vi "Updater Convert TDMS Test Runs 4.3 to 5.0 PIM.vi"(7 "Source TDMS File In":refnum<k34>, 8 "error in (no error)":errorcluster, 10 "Group Name In":string, 11 "New TDMS File In":refnum<k34>) -> (0 "error out":errorcluster, 2 "Group Name Out":string, 3 "New TDMS File Out":refnum<k34>, 5 "Source TDMS File Out":refnum<k34>)   [LabVIEW 2011]
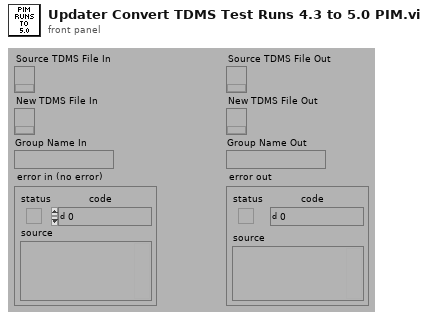
[diagram p1: front panel]
types:
  T1 = typedef "PIM Channel Type.ctl" = enum16{"Invalid", "Frequency", "Power", "CheckTx", "Unleveled", "Squelch", "Time", "Ref Limit", "IM Overload", "IM Power", "IM Frequency"}
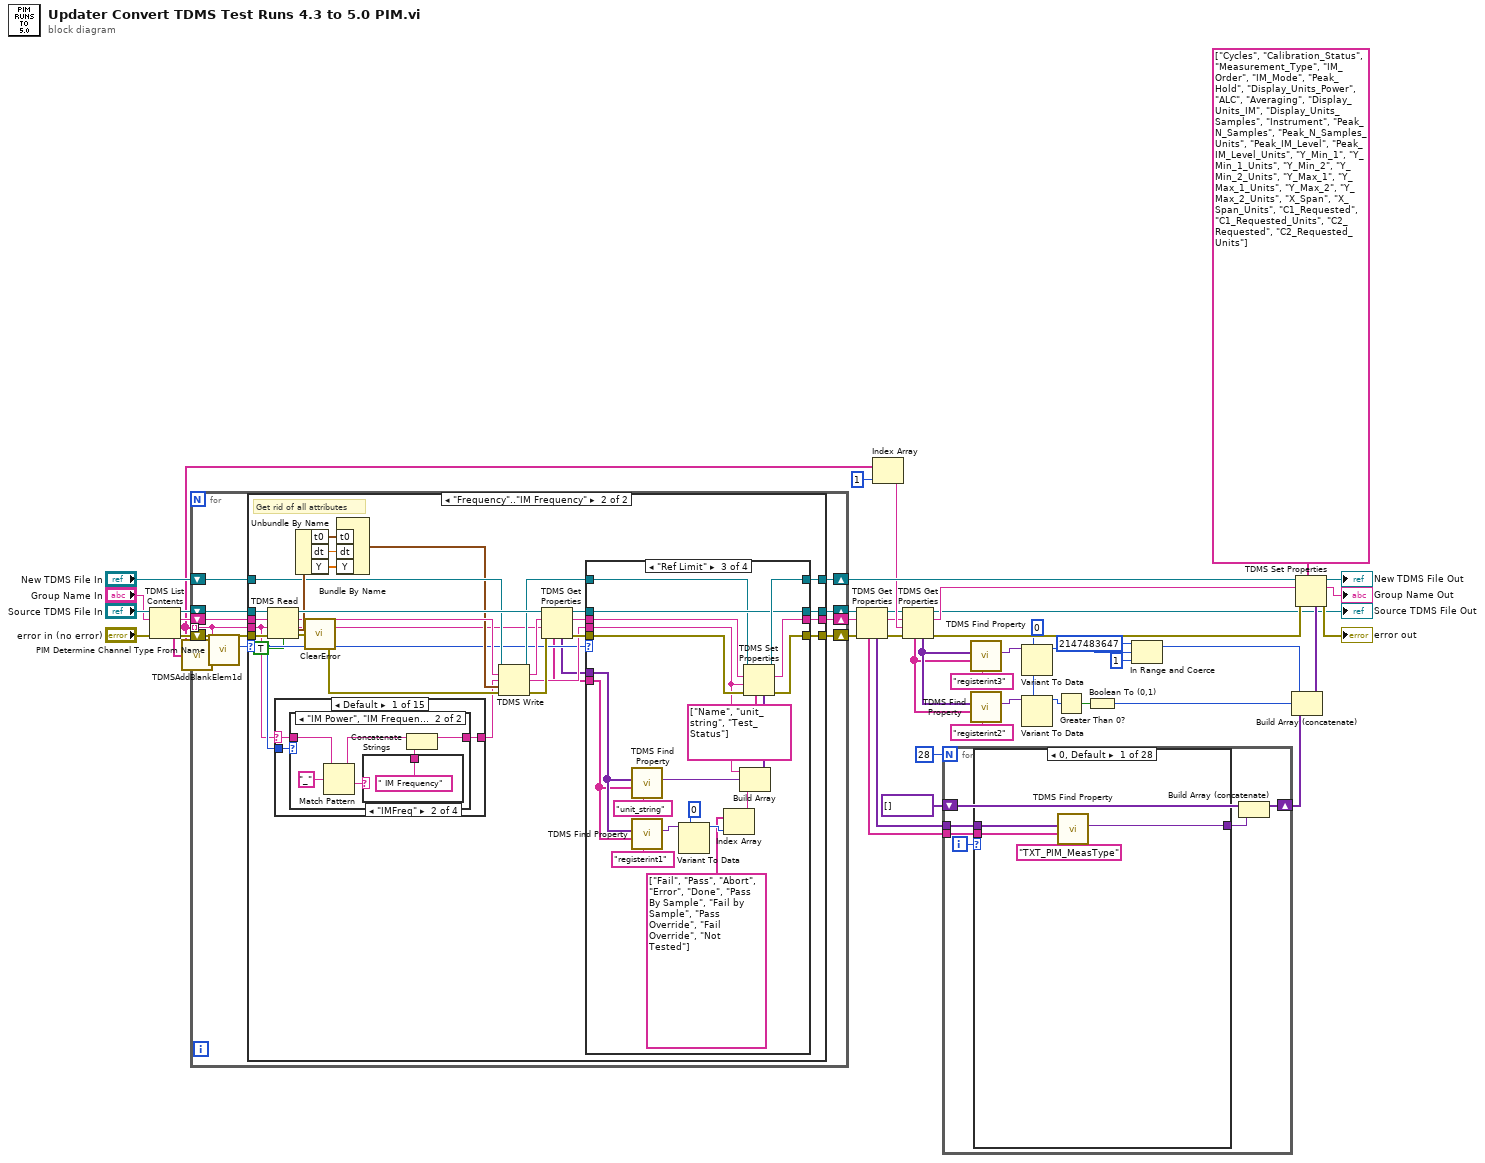
[diagram p0: block diagram]
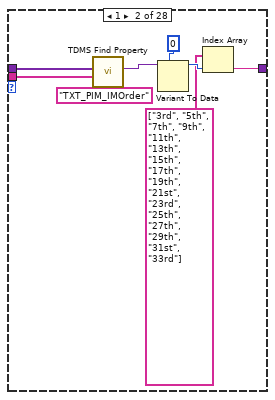
[diagram p2: hidden frame]
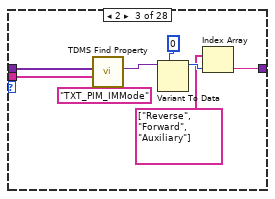
[diagram p3: hidden frame]
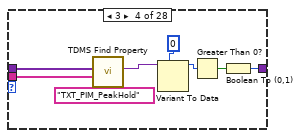
[diagram p4: hidden frame]
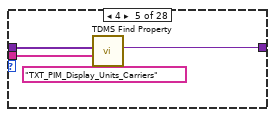
[diagram p5: hidden frame]
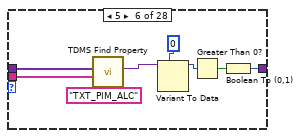
[diagram p6: hidden frame]
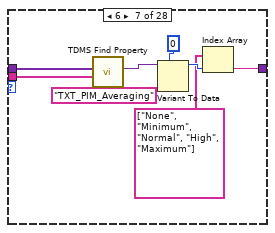
[diagram p7: hidden frame]
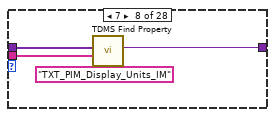
[diagram p8: hidden frame]
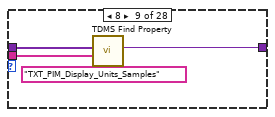
[diagram p9: hidden frame]
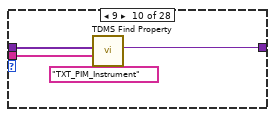
[diagram p10: hidden frame]
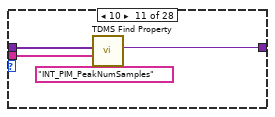
[diagram p11: hidden frame]
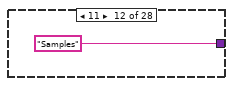
[diagram p12: hidden frame]
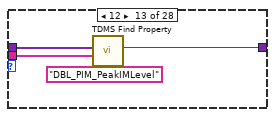
[diagram p13: hidden frame]
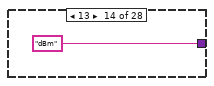
[diagram p14: hidden frame]
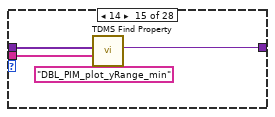
[diagram p15: hidden frame]
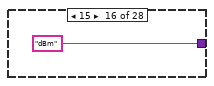
[diagram p16: hidden frame]
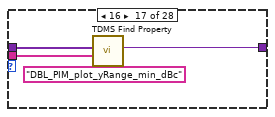
[diagram p17: hidden frame]
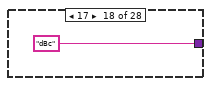
[diagram p18: hidden frame]
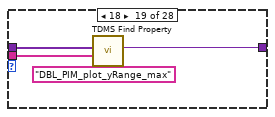
[diagram p19: hidden frame]
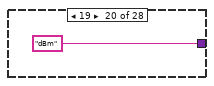
[diagram p20: hidden frame]
diagram:
  w18 = 0
  n1 = TDMS List Contents(4:"error in (no error)", 6:"Group Name In", 7:"Source TDMS File In") -> (0:w42:errorcluster, 1:w1:string[], 2:w40:string, 3:w41:refnum<k34>)
  n2 = call <vilib>:"TDMSAddBlankElem1d.vi"("input string array"=w1) -> ("output string array with blank element at the beginning"=w14:string[])
  n3 = for {
    shift-right: [w54] -> w11
    shift-left: w42 -> [w51]
    shift-right: [w55] -> w12
    shift-left: w41 -> [w50]
    tunnel: w14 -> [w48] mode=indexing
    shift-right: [w53] -> w10
    shift-left: w40 -> [w49]
    shift-right: [w52] -> w30
    shift-left: "New TDMS File In" -> [w47]
    n4 = call "PIM Determine Channel Type From Name.vi"("Channel Name"=w48) -> ("Channel Type"=w46:T1)  [unwired: 10 out]
    n5 = case shown="\"Frequency\"..\"IM Frequency\"" w46 {
      selector: w46 -> [_ w66]
      tunnel: [w59 w90] -> w55
      tunnel: [w56 w89] -> w54
      tunnel: [w58 w88] -> w53
      tunnel: [w57 w87] -> w52
      tunnel: w51 -> [w56 w83]
      tunnel: w50 -> [w59 w81]
      tunnel: w49 -> [w58 w80]
      tunnel: w48 -> [_ w65]
      tunnel: w47 -> [w57 w75]
      frame "Invalid" {
        # "Empty channel for Group level."
      }
      frame "Frequency".."IM Frequency" {
        # "Get rid of all attributes"
        n6 = TDMS Read(0:w81, 5:w80, 7:w65, 11:w83, 13:TRUE ("return channels in file order? (F)")) -> (4:w82:refnum<k34>, 6:w73:string, 8:w68:string, 10:w79:waveform(dbl), 15:w61:errorcluster)  [unwired: 3 in, 1 out]
        n7 = case shown="Default" w65 {
          selector: w65 -> [w92 _ _ _ _ _ _ _ _ _ _ _ _ _ _]
          tunnel: [w91 "Tx1 Frequency" "Tx1 Power" "Tx1 CheckTx" "Tx1 Unleveled" "Tx1 Squelch" "Tx2 Frequency" "Tx2 Power" "Tx2 CheckTx" "Tx2 Unleveled" "Tx2 Squelch" "Elapsed Time" "Ref Limit 1" "Ref Limit 2" "IM Overload"] -> w64
          tunnel: w66 -> [w93 _ _ _ _ _ _ _ _ _ _ _ _ _ _]
          frame Default {
            n8 = case shown="\"IM Power\", \"IM Frequency\"" w93 {
              tunnel: w92 -> [w94 w99]
              tunnel: [w94 w95] -> w91
              frame Default {
              }
              frame "IM Power", "IM Frequency" {
                n9 = Match Pattern(string=w99, regular expression="_") -> (before substring=w98:string, after substring=w97:string)  [unwired: 3 out]
                n10 = case shown="\"IMFreq\"" w97 {
                  tunnel: [_ " IM Frequency" " IM Power 1" " IM Power 2"] -> w96
                  frame Default {
                  }
                  frame "IMFreq" {
                  }
                  frame "IMPower" {
                  }
                  frame "IMPowerdBc" {
                  }
                }
                n11 = Concatenate Strings(w98, w96) -> (w95:string)
              }
            }
          }
          frame "Tx1Frequency" {
          }
          frame "Tx1Power" {
          }
          frame "Tx1CheckTx" {
          }
          frame "Tx1Unleveled" {
          }
          frame "Tx1Squelch" {
          }
          frame "Tx2Frequency" {
          }
          frame "Tx2Power" {
          }
          frame "Tx2CheckTx" {
          }
          frame "Tx2Unleveled" {
          }
          frame "Tx2Squelch" {
          }
          frame "elapsed_time" {
          }
          frame "RefLimit" {
          }
          frame "RefLimitdBc" {
          }
          frame "IMOverload" {
          }
        }
        n12 = Unbundle By Name(w79) -> ("t0"=w78:timestamp, "dt"=w77:dbl, "Y"=w76:dbl[])
        n13 = call <vilib>:"ClearError.vi"("error in (no error)"=w61) -> ("error out"=w74:errorcluster)
        n14 = Bundle By Name("t0"=w78, "dt"=w77, "Y"=w76) -> (w69:waveform(dbl))  [unwired: 1 out]
        n15 = TDMS Write(0:w75, 5:w73, 7:w64, 9:w69, 11:w74) -> (4:w70:refnum<k34>, 6:w72:string, 8:w67:string, 15:w71:errorcluster)  [unwired: 1 in]
        n16 = TDMS Get Properties(8:w71, 9:w68, 10:w72, 11:w82) -> (0:w86:errorcluster, 2:w85:string, 3:w84:refnum<k34>, 4:w63:variant[], 6:w62:string[])  [unwired: 3 out]
        n17 = case shown="\"Ref Limit\"" w66 {
          tunnel: w86 -> [w120 w124 w146 w158]
          tunnel: w85 -> [w119 w125 w147 w159]
          tunnel: w84 -> [w121 w130 w150 w161]
          tunnel: [w121 w130 w150 w161] -> w90
          tunnel: [w120 w133 w153 w162] -> w89
          tunnel: w67 -> [_ w122 w144 w157]
          tunnel: [w119 w134 w154 w163] -> w88
          tunnel: w70 -> [w118 w126 w148 w160]
          tunnel: [w118 w135 w155 w164] -> w87
          tunnel: w62 -> [_ w127 w141 _]
          tunnel: w63 -> [_ w128 w142 _]
          frame "Invalid" {
          }
          frame "Frequency", "Power", "Time", "IM Power", "IM Frequency" {
            n18 = call "TDMS Find Property.vi"("Property Name"="unit_string", "Property Names"=w127, "Property Values"=w128) -> ("Property Value"=w123:variant)  [unwired: 5 out]
            n19 = Build Array(w122, w123) -> (w131:variant[])
            n20 = TDMS Set Properties(5:w131, 7:string[] ["Name", "unit_string"], 8:w124, 9:w122, 10:w125, 11:w126) -> (0:w133:errorcluster, 2:w134:string, 3:w135:refnum<k34>)  [unwired: 1 out]
          }
          frame "Ref Limit" {
            n21 = call "TDMS Find Property.vi"("Property Name"="unit_string", "Property Names"=w141, "Property Values"=w142) -> ("Property Value"=w145:variant)  [unwired: 5 out]
            n22 = call "TDMS Find Property.vi"("Property Name"="registerint1", "Property Names"=w141, "Property Values"=w142) -> ("Property Value"=w137:variant)  [unwired: 5 out]
            n23 = Variant To Data(type=0, Variant=w137) -> (data=w140:i32)  [unwired: 1 in, 1 out]
            n24 = Index Array(array=string[] ["Fail", "Pass", "Abort", "Error", "Done", "Pass By Sample", "Fail by Sample", "Pass Override", "Fail Override", "Not Tested"], index=w140) -> (element=w136:string)
            n25 = Build Array(w144, w145, w136) -> (w151:variant[])
            n26 = TDMS Set Properties(5:w151, 7:string[] ["Name", "unit_string", "Test_Status"], 8:w146, 9:w144, 10:w147, 11:w148) -> (0:w153:errorcluster, 2:w154:string, 3:w155:refnum<k34>)  [unwired: 1 out]
          }
          frame "CheckTx".."Squelch", "IM Overload" {
            n27 = TDMS Set Properties(5:w157, 7:"Name", 8:w158, 9:w157, 10:w159, 11:w160) -> (0:w162:errorcluster, 2:w163:string, 3:w164:refnum<k34>)  [unwired: 1 out]
          }
        }
      }
    }
  }
  n28 = TDMS Get Properties(8:w11, 10:w10, 11:w12) -> (0:w8:errorcluster, 2:w7:string, 3:w9:refnum<k34>, 4:w4:variant[], 6:w3:string[])  [unwired: 1 in, 3 out]
  n29 = Index Array(array=w14, index=1) -> (element=w13:string)
  n30 = TDMS Get Properties(8:w8, 9:w13, 10:w7, 11:w9) -> (0:w39:errorcluster, 2:w36:string, 3:→"Source TDMS File Out":refnum<k34>, 4:w21:variant[], 6:w20:string[])  [unwired: 1 in, 2 out]
  n31 = for {
    N: 28 -> [_]
    shift-right: [w165] -> w2
    shift-left: variant[] [] ("appended array") -> [w166]
    tunnel: w4 -> [w169]
    tunnel: w3 -> [w168]
    i -> [w170]
    n32 = case shown="0, Default" w170 {
      tunnel: w169 -> [w173 w181 w189 w197 w201 w209 w217 w221 w225 w229 w233 _ w238 _ w243 _ w248 _ w253 _ w258 _ w263 _ w268 _ w273 _]
      tunnel: w168 -> [w172 w180 w188 w196 w200 w208 w216 w220 w224 w228 w232 _ w237 _ w242 _ w247 _ w252 _ w257 _ w262 _ w267 _ w272 _]
      tunnel: [w171 w175 w183 w192 w199 w204 w211 w219 w223 w227 w231 "Samples" w236 "dBm" w241 "dBm" w246 "dBc" w251 "dBm" w256 "dBc" w261 "MHz" w266 "dBm" w271 "dBm"] -> w167
      frame 0, Default {
        n33 = call "TDMS Find Property.vi"("Property Name"="TXT_PIM_MeasType", "Property Names"=w172, "Property Values"=w173) -> ("Property Value"=w171:variant)  [unwired: 5 out]
      }
      frame 1 {
        n34 = call "TDMS Find Property.vi"("Property Name"="TXT_PIM_IMOrder", "Property Names"=w180, "Property Values"=w181) -> ("Property Value"=w178:variant)  [unwired: 5 out]
        n35 = Variant To Data(type=0, Variant=w178) -> (data=w177:i32)  [unwired: 1 in, 1 out]
        n36 = Index Array(array=string[] ["3rd", "5th", "7th", "9th", "11th", "13th", "15th", "17th", "19th", "21st", "23rd", "25th", "27th", "29th", "31st", "33rd"], index=w177) -> (element=w175:string)
      }
      frame 2 {
        n37 = call "TDMS Find Property.vi"("Property Name"="TXT_PIM_IMMode", "Property Names"=w188, "Property Values"=w189) -> ("Property Value"=w186:variant)  [unwired: 5 out]
        n38 = Variant To Data(type=0, Variant=w186) -> (data=w185:i32)  [unwired: 1 in, 1 out]
        n39 = Index Array(array=string[] ["Reverse", "Forward", "Auxiliary"], index=w185) -> (element=w183:string)
      }
      frame 3 {
        n40 = call "TDMS Find Property.vi"("Property Name"="TXT_PIM_PeakHold", "Property Names"=w196, "Property Values"=w197) -> ("Property Value"=w194:variant)  [unwired: 5 out]
        n41 = Variant To Data(type=0, Variant=w194) -> (data=w191:i32)  [unwired: 1 in, 1 out]
        n42 = Greater Than 0?(x=w191) -> (x > 0?=w193:bool)
        n43 = Boolean To (0,1)(Boolean=w193) -> (0, 1=w192:i16)
      }
      frame 4 {
        n44 = call "TDMS Find Property.vi"("Property Name"="TXT_PIM_Display_Units_Carriers", "Property Names"=w200, "Property Values"=w201) -> ("Property Value"=w199:variant)  [unwired: 5 out]
      }
      frame 5 {
        n45 = call "TDMS Find Property.vi"("Property Name"="TXT_PIM_ALC", "Property Names"=w208, "Property Values"=w209) -> ("Property Value"=w206:variant)  [unwired: 5 out]
        n46 = Variant To Data(type=0, Variant=w206) -> (data=w203:i32)  [unwired: 1 in, 1 out]
        n47 = Greater Than 0?(x=w203) -> (x > 0?=w205:bool)
        n48 = Boolean To (0,1)(Boolean=w205) -> (0, 1=w204:i16)
      }
      frame 6 {
        n49 = call "TDMS Find Property.vi"("Property Name"="TXT_PIM_Averaging", "Property Names"=w216, "Property Values"=w217) -> ("Property Value"=w214:variant)  [unwired: 5 out]
        n50 = Variant To Data(type=0, Variant=w214) -> (data=w213:i32)  [unwired: 1 in, 1 out]
        n51 = Index Array(array=string[] ["None", "Minimum", "Normal", "High", "Maximum"], index=w213) -> (element=w211:string)
      }
      frame 7 {
        n52 = call "TDMS Find Property.vi"("Property Name"="TXT_PIM_Display_Units_IM", "Property Names"=w220, "Property Values"=w221) -> ("Property Value"=w219:variant)  [unwired: 5 out]
      }
      frame 8 {
        n53 = call "TDMS Find Property.vi"("Property Name"="TXT_PIM_Display_Units_Samples", "Property Names"=w224, "Property Values"=w225) -> ("Property Value"=w223:variant)  [unwired: 5 out]
      }
      frame 9 {
        n54 = call "TDMS Find Property.vi"("Property Name"="TXT_PIM_Instrument", "Property Names"=w228, "Property Values"=w229) -> ("Property Value"=w227:variant)  [unwired: 5 out]
      }
      frame 10 {
        n55 = call "TDMS Find Property.vi"("Property Name"="INT_PIM_PeakNumSamples", "Property Names"=w232, "Property Values"=w233) -> ("Property Value"=w231:variant)  [unwired: 5 out]
      }
      frame 11 {
      }
      frame 12 {
        n56 = call "TDMS Find Property.vi"("Property Name"="DBL_PIM_PeakIMLevel", "Property Names"=w237, "Property Values"=w238) -> ("Property Value"=w236:variant)  [unwired: 5 out]
      }
      frame 13 {
      }
      frame 14 {
        n57 = call "TDMS Find Property.vi"("Property Name"="DBL_PIM_plot_yRange_min", "Property Names"=w242, "Property Values"=w243) -> ("Property Value"=w241:variant)  [unwired: 5 out]
      }
      frame 15 {
      }
      frame 16 {
        n58 = call "TDMS Find Property.vi"("Property Name"="DBL_PIM_plot_yRange_min_dBc", "Property Names"=w247, "Property Values"=w248) -> ("Property Value"=w246:variant)  [unwired: 5 out]
      }
      frame 17 {
      }
      frame 18 {
        n59 = call "TDMS Find Property.vi"("Property Name"="DBL_PIM_plot_yRange_max", "Property Names"=w252, "Property Values"=w253) -> ("Property Value"=w251:variant)  [unwired: 5 out]
      }
      frame 19 {
      }
      frame 20 {
        n60 = call "TDMS Find Property.vi"("Property Name"="DBL_PIM_plot_yRange_max_dBc", "Property Names"=w257, "Property Values"=w258) -> ("Property Value"=w256:variant)  [unwired: 5 out]
      }
      frame 21 {
      }
      frame 22 {
        n61 = call "TDMS Find Property.vi"("Property Name"="DBL_PIM_plot_xRange_span", "Property Names"=w262, "Property Values"=w263) -> ("Property Value"=w261:variant)  [unwired: 5 out]
      }
      frame 23 {
      }
      frame 24 {
        n62 = call "TDMS Find Property.vi"("Property Name"="DBL_PIM_C1_Requested_dBm", "Property Names"=w267, "Property Values"=w268) -> ("Property Value"=w266:variant)  [unwired: 5 out]
      }
      frame 25 {
      }
      frame 26 {
        n63 = call "TDMS Find Property.vi"("Property Name"="DBL_PIM_C2_Requested_dBm", "Property Names"=w272, "Property Values"=w273) -> ("Property Value"=w271:variant)  [unwired: 5 out]
      }
      frame 27 {
      }
    }
    n64 = Build Array (concatenate)(w166, w167) -> (w165:variant[])
  }
  n65 = call "TDMS Find Property.vi"("Property Name"="registerint3", "Property Names"=w20, "Property Values"=w21) -> ("Property Value"=w28:variant)  [unwired: 5 out]
  n66 = call "TDMS Find Property.vi"("Property Name"="registerint2", "Property Names"=w20, "Property Values"=w21) -> ("Property Value"=w19:variant)  [unwired: 5 out]
  n67 = Variant To Data(type=w18, Variant=w28) -> (data=w27:i32)  [unwired: 1 in, 1 out]
  n68 = Variant To Data(type=w18, Variant=w19) -> (data=w17:i32)  [unwired: 1 in, 1 out]
  n69 = Greater Than 0?(x=w17) -> (x > 0?=w16:bool)
  n70 = Boolean To (0,1)(Boolean=w16) -> (0, 1=w23:i16)
  n71 = In Range and Coerce(upper limit=2147483647, x=w27, lower limit=1) -> (coerced(x)=w26:i32)  [unwired: 1 out]
  n72 = Build Array (concatenate)(w26, w23, w2) -> (w37:variant[])
  n73 = TDMS Set Properties(5:w37, 7:string[] ["Cycles", "Calibration_Status", "Measurement_Type", "IM_Order", "IM_Mode", "Peak_Hold", "Display_Units_Power", "ALC", "Averaging", "Display_Units_IM", "Display_Units_Samples", "Instrument", "Peak_N_Samples", "Peak_N_Samples_Units", "Peak_IM_Level", "Peak_IM_Level_Units", "Y_Min_1", "Y_Min_1_Units", "Y_Min_2", "Y_Min_2_Units", "Y_Max_1", "Y_Max_1_Units", "Y_Max_2", "Y_Max_2_Units", "X_Span", "X_Span_Units", "C1_Requested", "C1_Requested_Units", "C2_Requested", "C2_Requested_Units"], 8:w39, 10:w36, 11:w30) -> (0:→"error out":errorcluster, 2:→"Group Name Out":string, 3:→"New TDMS File Out":refnum<k34>)  [unwired: 2 out]
